vi "GUI_StagingDelayStage.vi"() -> ()   [LabVIEW 2013]
uses:
  shared programs/GUI_Template/GUI_master/tcp new data cluster.ctl
panel:
  out "XY Graph":cluster{dbl[], dbl[]}(graph)
  out "Position.Axis 3::1 3":dbl(graph) caption="position.Axis 3"
  in  "time::2":dbl caption="position.Axis 3" min=-100000.0 max=100000.0 format="%#_12g"
  in  "GUIdevice 2":string="TapeDrive"
  out "Position.Axis 3::1 2":dbl(graph) caption="position.Axis 3"
  in  "Position.Axis 3::1":dbl caption="position.Axis 3" min=0.0 max=50.0 format="%#_12g"
  in  "stop":bool
  in  "GUIdevice 1":string="TapeDrive"
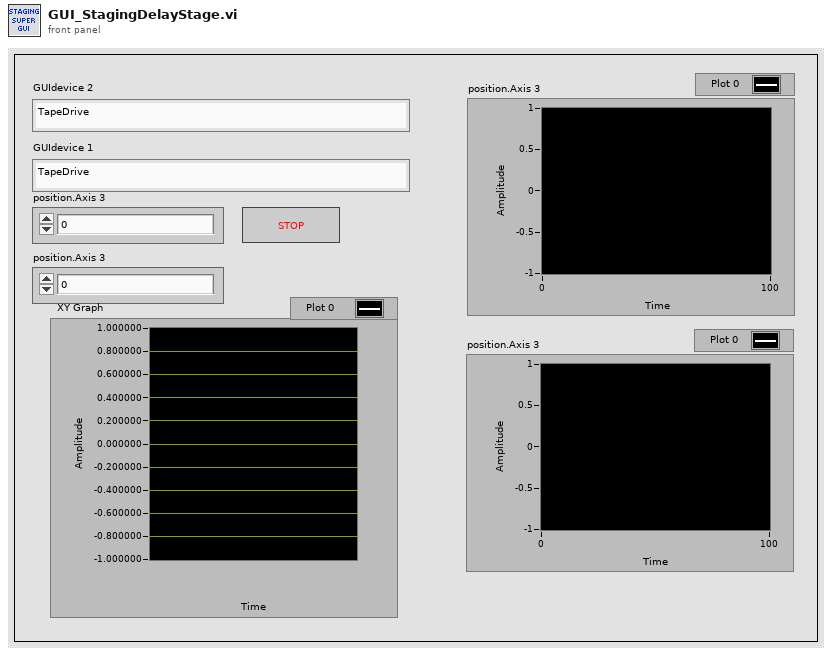
[diagram p1: front panel]
types:
  T1 = typedef "tcp new data cluster.ctl" = cluster{"EventEnum":enum16{"new data", "connection status update"}, "Device name":string}
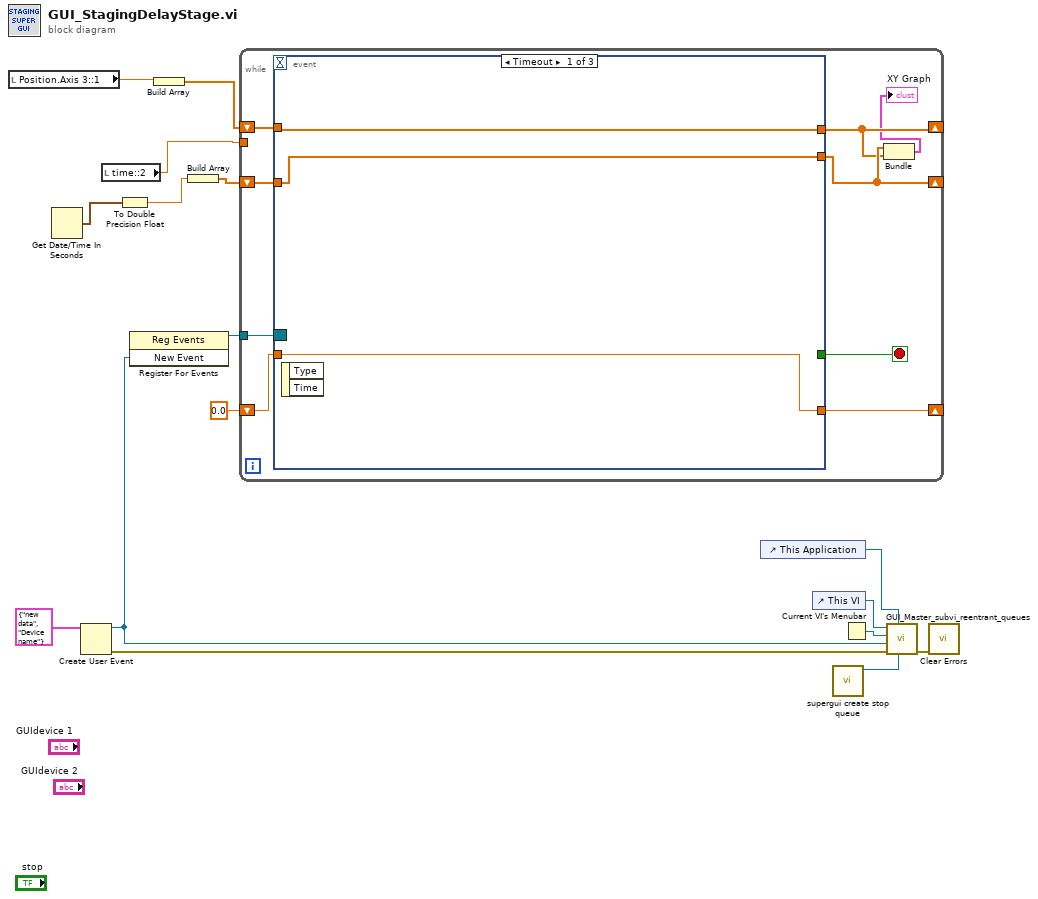
[diagram p0: block diagram]
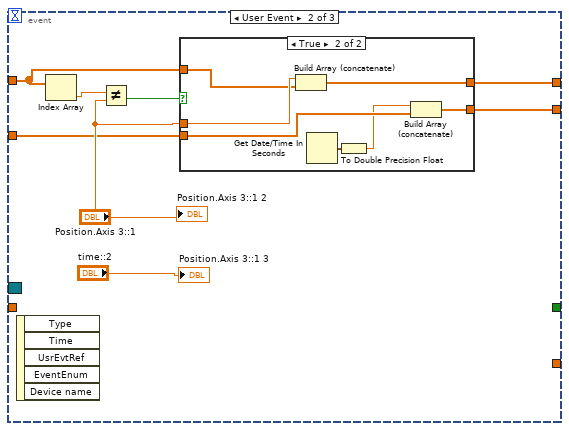
[diagram p2: hidden frame]
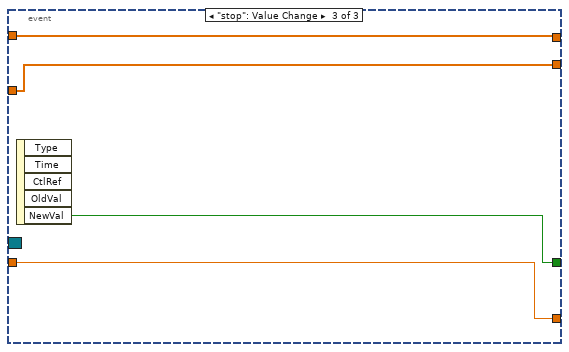
[diagram p4: hidden frame]
diagram:
  n1 = local read "Position.Axis 3::1"() -> (w7:dbl)
  n2 = Get Date/Time In Seconds() -> (seconds since 1Jan1904=w3:timestamp)
  n3 = Create User Event(user event datatype=T1 {"EventEnum"=enum."new data", "Device name"="Device name"} ("New Event")) -> (user event=w13:refnum<user-event>, error out=w15:errorcluster)  [unwired: 1 in]
  n4 = local read "time::2"() -> (w5:dbl)
  n5 = To Double Precision Float(number=w3) -> (double precision float=w2:dbl)
  n6 = register-events(w13) -> (reference out=w12:refnum<event-registration>)  [unwired: 2 in, 1 out]
  n7 = Build Array(w7) -> (w6:dbl[])
  n8 = Build Array(w2) -> (w4:dbl[])
  n9 = while {
    tunnel: w12 -> [w25]
    shift-right: [w22] -> _
    shift-left: 0.0 -> [w23]
    shift-right: [w18] -> _
    shift-left: w6 -> [w21]
    shift-right: [w19] -> _
    shift-left: w4 -> [w20]
    tunnel: w5 -> [_]
    stop <- w24 stop-if-true
    n10 = event shown="[0] Timeout" {
      selector: w25 -> [_ _ _]
      dyn-events: _ -> [_ _ _]
      timeout: _ -> [_ _ _]
      tunnel: [_ _ w49] -> w24
      tunnel: w23 -> [w28 _ w48]
      tunnel: [w28 _ w48] -> w22
      tunnel: w21 -> [w27 w33 w47]
      tunnel: [w27 w32 w47] -> w18
      tunnel: [w26 w31 w46] -> w19
      tunnel: w20 -> [w26 w30 w46]
      event Timeout {
        n11 = event-data() -> ()  [unwired: 1 in, 2 out]
      }
      event User Event {
        n12 = event-data() -> ()  [unwired: 1 in, 5 out]
        n13 = Index Array(array=w33) -> (element=w34:dbl)  [unwired: 1 in]
        n14 = Not Equal?(x=w34, y="Position.Axis 3::1") -> (x != y?=w29:bool)
        n15 = case shown="True" w29 {
          tunnel: "Position.Axis 3::1" -> [_ w45]
          tunnel: w33 -> [w38 w44]
          tunnel: [w38 w43] -> w32
          tunnel: [w37 w42] -> w31
          tunnel: w30 -> [w37 w41]
          frame False {
          }
          frame True {
            n16 = Build Array (concatenate)(w45, w44) -> (w43:dbl[])
            n17 = Get Date/Time In Seconds() -> (seconds since 1Jan1904=w40:timestamp)
            n18 = To Double Precision Float(number=w40) -> (double precision float=w39:dbl)
            n19 = Build Array (concatenate)(w39, w41) -> (w42:dbl[])
          }
        }
        "Position.Axis 3::1 2" <- "Position.Axis 3::1"
        "Position.Axis 3::1 3" <- "time::2"
      }
      event "stop": Value Change {
        n20 = event-data() -> ("NewVal"=w49:bool)  [unwired: 1 in, 4 out]
      }
    }
    n21 = Bundle(w19, w18) -> (→"XY Graph":cluster{dbl[], dbl[]})  [unwired: 1 in]
  }
  n22 = control-ref of="This Application"() -> (w8:refnum<vi>)
  n23 = control-ref of="This VI"() -> (w10:refnum<vi>)
  n24 = call "supergui create stop queue.vi"() -> ("STOP Queue out"=w1:refnum<queue>)  [unwired: 11 in]
  n25 = Current VI's Menubar() -> (w9:refnum<k9>)
  n26 = call "GUI_Master_subvi_reentrant_queues.vi"("STOP Queue in"=w1, "This Application"=w8, "error in (no error)"=w15, "tcp data event"=w13, "Caller menu reference"=w9, "Caller VI ref"=w10) -> ("error out"=w14:errorcluster)  [unwired: 5 in]
  n27 = call <vilib>:"Clear Errors.vi"("error in (no error)"=w14) -> ()  [unwired: 6 in, 1 out]
